vi "UHR-Fleezers Control (host) -Leonardo 04-2018 V1.vi"(0 "Tab Control":T5(tab)=enum."Trap Control (RF)") -> ()   [LabVIEW 2013] (continued)
              tunnel: w2073 -> [_ w2136]
              tunnel: w2071 -> [_ w2135]
              frame False {
              }
              frame True {
                w2131 = FALSE ("Get Point")
                n1369 = local read "Scan lines (y)"() -> (w2140:u64)
                n1370 = local read "Actual MCL Inc (V)"() -> (w2132:dbl)
                n1371 = local read "Scan steps (MCL)"() -> (w2139:u64)
                n1372 = Divide "Y Pix/step"(x=w2135, y=w2140) -> (x/y=w2147:dbl)
                n1373 = Divide "Y V/pix"(x=w2132, y=w2147) -> (x/y=w2146:dbl)
                n1374 = Divide "Y half step offset"(x=w2132, y=2.0) -> (x/y=w2148:dbl)
                n1375 = Divide "X pix/step"(x=w2136, y=w2139) -> (x/y=w2145:dbl)
                n1376 = Negate(x=w2148) -> (-x=w2149:dbl)
                n1377 = local read "Initial Y"() -> (w2155:dbl)
                n1378 = Multiply(x=w2137, y=w2146) -> (x*y=w2156:dbl)
                n1379 = Divide "X half step offset"(x=w2132, y=2.0) -> (x/y=w2142:dbl)
                n1380 = Divide "X V/pix"(x=w2132, y=w2145) -> (x/y=w2144:dbl)
                n1381 = Multiply(x=w2132, y=w2139) -> (x*y=w2151:dbl)
                n1382 = Compound Arithmetic op=ADD(w2149, w2156, w2155) -> (w2133:dbl)
                "Pointer Y (V)" <- w2133
                n1383 = Multiply(x=w2144, y=w2138) -> (x*y=w2153:dbl)
                n1384 = Negate(x=w2142) -> (-x=w2141:dbl)
                n1385 = local read "Initial X"() -> (w2154:dbl)
                n1386 = Negate(x=w2153) -> (-x=w2152:dbl)
                n1387 = Compound Arithmetic op=ADD(w2141, w2151, w2154, w2152) -> (w2134:dbl)
                "Pointer X (V)" <- w2134
                n1388 = Or(x="Set X Only", y="Set Confocal Spot (X-Y)") -> (x .or. y?=w2127:bool)
                n1389 = Or(x="Set Confocal Spot (X-Y)", y="Set Y Only") -> (x .or. y?=w2126:bool)
                n1390 = case shown="True" w2127 {
                  tunnel: w2134 -> [_ w2157]
                  frame False {
                  }
                  frame True {
                    n1391 = property on="AO2" class="Slide (strict)"("Val(Sgnl)"=w2157) -> ()  [unwired: 2 in, 2 out]
                  }
                }
                n1392 = case shown="True" w2126 {
                  tunnel: w2133 -> [_ w2158]
                  frame False {
                  }
                  frame True {
                    n1393 = property on="AO1" class="Slide (strict)"("Val(Sgnl)"=w2158) -> ()  [unwired: 2 in, 2 out]
                  }
                }
                n1394 = local write "Set Confocal Spot (X-Y)"(w2131) -> ()
                n1395 = local write "Set X Only"(w2131) -> ()
                n1396 = local write "Set Y Only"(w2131) -> ()
              }
            }
          }
          frame 3 {
            n1397 = local read "BD 2 Frequency 1 (MHz)"() -> (w2159:dbl)
            n1398 = local read "BD 1 Frequency 1 (MHz)"() -> (w2160:dbl)
            n1399 = local write "Manipulating Trap"(TRUE ("Manipulating Trap")) -> ()
            n1400 = local write "Coords"(T8 {"Horizontal"=0, "Vertical"=0} ("Coords")) -> ()
            n1401 = while {
              tunnel: w2165 -> [w2170]
              tunnel: w2163 -> [w2169]
              tunnel: w2161 -> [w2168]
              tunnel: w2160 -> [w2167]
              tunnel: w2159 -> [w2166]
              stop <- w2171 stop-if-true
              n1402 = event shown="[0] \"Pane\": Mouse Move" {
                selector: _ -> [_ _]
                dyn-events: _ -> [_ _]
                timeout: _ -> [_ _]
                tunnel: ["Force Manip Abort" w2235] -> w2171
                tunnel: w2170 -> [w2178 _]
                tunnel: w2169 -> [w2176 _]
                tunnel: w2168 -> [w2175 _]
                tunnel: w2167 -> [w2174 _]
                tunnel: w2166 -> [w2173 _]
                event Mouse Move {
                  n1403 = event-data() -> ("Time"=w2179:u32, "Coords"=w2180:T8)  [unwired: 3 out]
                  n1404 = Less?(x=w2179, y=w2178) -> (x < y?=w2177:bool)
                  n1405 = case "Makes sure old motion events prior to mouse click aren't used" shown="False" w2177 {
                    tunnel: w2180 -> [w2222 _]
                    tunnel: w2176 -> [w2223 _]
                    tunnel: w2175 -> [w2200 _]
                    tunnel: w2174 -> [w2196 _]
                    tunnel: w2173 -> [w2195 _]
                    frame False {
                      n1406 = Subtract(x=w2222, y=w2223) -> (x-y=w2221:T8)
                      "Coords" <- w2221
                      n1407 = local read "Y RF Frequency Limits (MHz)"() -> (w2181:T16)
                      n1408 = To Double Precision Float(number=w2221) -> (double precision float=w2220:cluster{"Horizontal":dbl, "Vertical":dbl})
                      n1409 = Multiply(x=cluster{"Horizontal":dbl, "Vertical":dbl} {"Horizontal"=-1.0, "Vertical"=1.0}, y="Manipulation Scaling") -> (x*y=w2216:cluster{"Horizontal":dbl, "Vertical":dbl})
                      n1410 = local read "X RF Frequency Limits (MHz)"() -> (w2182:T16)
                      n1411 = Multiply(x=w2220, y=w2216) -> (x*y=w2218:cluster{"Horizontal":dbl, "Vertical":dbl})
                      n1412 = Unbundle By Name(w2218) -> ("Horizontal"=w2213:dbl, "Vertical"=w2217:dbl)
                      n1413 = Unbundle By Name(w2181) -> ("Maximum"=w2184:dbl, "Minimum"=w2183:dbl)
                      n1414 = Boolean To (0,1)(Boolean="Manip. X?") -> (0, 1=w2211:i16)
                      n1415 = Boolean To (0,1)(Boolean="Manip. Y?") -> (0, 1=w2208:i16)
                      n1416 = local read "BD 1 Frequency 2 (MHz)"() -> (w2198:dbl)
                      n1417 = Multiply(x=w2217, y=w2208) -> (x*y=w2210:dbl)
                      n1418 = Multiply(x=w2211, y=w2213) -> (x*y=w2214:dbl)
                      n1419 = local read "BD 2 Frequency 2 (MHz)"() -> (w2197:dbl)
                      n1420 = Unbundle By Name(w2182) -> ("Maximum"=w2186:dbl, "Minimum"=w2185:dbl)
                      n1421 = Add(x=w2195, y=w2210) -> (x+y=w2188:dbl)
                      n1422 = Add(x=w2196, y=w2214) -> (x+y=w2190:dbl)
                      n1423 = In Range and Coerce(upper limit=w2186, x=w2190, lower limit=w2185) -> (coerced(x)=w2189:dbl)  [unwired: 1 out]
                      n1424 = In Range and Coerce(upper limit=w2184, x=w2188, lower limit=w2183) -> (coerced(x)=w2187:dbl)  [unwired: 1 out]
                      n1425 = Subtract(x=w2189, y=w2198) -> (x-y=w2207:dbl)
                      n1426 = Subtract(x=w2187, y=w2197) -> (x-y=w2206:dbl)
                      n1427 = Square(x=w2207) -> (x^2=w2205:dbl)
                      n1428 = Square(x=w2206) -> (x^2=w2204:dbl)
                      n1429 = Add(x=w2205, y=w2204) -> (x+y=w2203:dbl)
                      n1430 = Square Root(x=w2203) -> (sqrt(x)=w2199:dbl)
                      n1431 = In Range and Coerce(upper limit="Limit Max (MHz)", x=w2199, lower limit="Limit Min (MHz)") -> (In Range?=w2192:bool)  [unwired: 1 out]
                      n1432 = Not(x="Limits Enable") -> (.not. x?=w2191:bool)
                      n1433 = Or(x=w2192, y=w2191) -> (x .or. y?=w2193:bool)
                      n1434 = case shown="True" w2193 {
                        tunnel: w2200 -> [_ w2233]
                        tunnel: w2199 -> [_ w2224]
                        tunnel: w2189 -> [_ w2231]
                        tunnel: w2198 -> [_ w2230]
                        tunnel: w2187 -> [_ w2229]
                        tunnel: w2197 -> [_ w2228]
                        tunnel: w2182 -> [_ w2226]
                        tunnel: w2181 -> [_ w2225]
                        frame False {
                        }
                        frame True {
                          n1435 = local read "BD 1 Frequency 3 (MHz)"() -> (w2232:dbl)
                          n1436 = local read "BD 2 Frequency 3 (MHz)"() -> (w2227:dbl)
                          n1437 = local write "Trap Delta (MHz)"(w2224) -> ()
                          n1438 = property on="Initial delta (MHz)" class="DigNum (strict)"("Val(Sgnl)"=w2224) -> ()  [unwired: 2 in, 2 out]
                          n1439 = call "set RF board frequency - interlace.vi"("Board 2 Frequency Limits"=w2225, "Board 1 Frequency Limits"=w2226, "FPGA VI Reference In"=w2233, "Board 2 Frequency 3 (MHz)"=w2227, "Board 1 Frequency 3 (MHz)"=w2232, "Board 2 Frequency 2 (MHz)"=w2228, "Board 2 Frequency 1 (MHz)"=w2229, "Board 1 Frequency 2 (MHz)"=w2230, "Board 1 Frequency 1  (MHz)"=w2231) -> ()  [unwired: 1 in, 2 out]
                          n1440 = local write "BD 2 Frequency 1 (MHz)"(w2229) -> ()
                          n1441 = local write "BD 1 Frequency 1 (MHz)"(w2231) -> ()
                        }
                      }
                    }
                    frame True {
                    }
                  }
                }
                event Mouse Up {
                  n1442 = event-data() -> ("Button"=w2234:u16)  [unwired: 8 out]
                  n1443 = case shown="3" w2234 {
                    tunnel: [FALSE TRUE] -> w2235
                    frame 0, Default {
                    }
                    frame 3 {
                      n1444 = local write "Manipulating Trap"(FALSE ("Manipulating Trap")) -> ()
                    }
                  }
                }
              }
            }
          }
        }
      }
      event Mouse Move {
        n1445 = event-data() -> ()  [unwired: 6 out]
      }
    }
    n1446 = local read "Stop All"() -> (w2056:bool)
    n1447 = node-c288() -> ()  [unwired: 2 out]
  }
  n1448 = node-c288(w51) -> ()  [unwired: 1 out]
  n1449 = node-c288(w101) -> ()  [unwired: 1 out]
  n1450 = node-c288(w108) -> ()  [unwired: 1 out]
  n1451 = node-c288(i64 1 ("Period"), 1 ("Processor")) -> (w194:T25)  [unwired: 2 out]
  n1452 = timed-loop "Acquire Data" {
    tunnel: w59 -> [w2544]
    tunnel: w75 -> [w2543]
    tunnel: [w2574] -> w68
    tunnel: [w2568] -> w67
    timing: w194 -> [_]
    timing-out: [_] -> w193
    tunnel: w92 -> [w2390]
    stop <- "Stop All" stop-if-true
    (unwired) u32 0 ("Number of Elements")
    w2377 = "NI_ChannelName" ("name")
    n1453 = node-c288() -> ()  [unwired: 2 out]
    n1454 = First Call?() -> (First Call?: T/F=w2343:bool)
    n1455 = Or(x="Reset", y=w2343) -> (x .or. y?=w2344:bool)
    n1456 = local read "MCL Tracking"() -> (w2281:bool)
    n1457 = case "Reset data stream" shown="True" w2344 {
      tunnel: w2544 -> [w2694 w2702]
      tunnel: w2543 -> [w2693 w2701]
      tunnel: [w2694 w2696] -> w2279
      tunnel: [w2693 w2695] -> w2539
      frame False {
      }
      frame True {
        w2699 = TRUE ("AI to FIFO")
        n1458 = local write "Overflow (data lost)"(FALSE ("Overflow (data lost)")) -> ()
        n1459 = call "reset FPGA DMA.vi"("error in"=w2701, "FPGA VI Reference In"=w2702) -> ("error out"=w2697:errorcluster, "FPGA VI Reference Out"=w2698:T20)
        n1460 = xnode "Read/Write Control"("FPGA VI Reference In"=w2698, "error in"=w2697, "AI to FIFO"=w2699, "APD to FIFO"=w2699) -> ("FPGA VI Reference Out"=w2696:T20, "error out"=w2695:errorcluster)
      }
    }
    n1461 = Or(x="Start AOD Scan", y="Trap Raster Scan") -> (x .or. y?=w2497:bool)
    n1462 = case "Start AOM raster scan" shown="True" w2497 {
      tunnel: w2279 -> [w3435 w3446]
      tunnel: w2539 -> [w3434 w3445]
      tunnel: [w3435 w3439] -> w2278
      tunnel: [w3434 w3438] -> w2538
      frame False {
      }
      frame True {
        n1463 = case shown="True" "Restart DMA? (AOD)" {
          tunnel: [w3486 w3488] -> w3440
          tunnel: [w3485 w3487] -> w3441
          tunnel: w3446 -> [w3486 w3490]
          tunnel: w3445 -> [w3485 w3489]
          frame False {
          }
          frame True {
            n1464 = local write "Overflow (data lost)"(FALSE ("Overflow (data lost)")) -> ()
            n1465 = call "reset FPGA DMA.vi"("error in"=w3489, "FPGA VI Reference In"=w3490) -> ("error out"=w3487:errorcluster, "FPGA VI Reference Out"=w3488:T20)
          }
        }
        n1466 = local write "Trap Raster Scan"(FALSE ("Trap Raster Scan")) -> ()
        n1467 = case shown="True" "Move MCL Also?" {
          tunnel: w3441 -> [w3450 w3480]
          tunnel: w3440 -> [w3451 w3481]
          tunnel: [w3449 w3484] -> w3439
          tunnel: [w3448 w3483] -> w3438
          tunnel: "Raster to target force?" -> [w3447 w3453]
          frame False {
            w3452 = TRUE ("AI to FIFO")
            n1468 = xnode "Read/Write Control"("FPGA VI Reference In"=w3451, "error in"=w3450, "AI to FIFO"=w3452, "APD to FIFO"=w3452, "Start scan"=w3452, "Raster to target force"=w3447) -> ("FPGA VI Reference Out"=w3449:T20, "error out"=w3448:errorcluster)
          }
          frame True {
            w3477 = FALSE ("1D or 2D Scan?")
            w3482 = TRUE ("AI to FIFO")
            # "Count for MCL loop"
            # "N total cycles"
            # "N steps"
            # "V_int"
            n1469 = local read "Scan Range (nm)"() -> (w3459:dbl)
            n1470 = local read "Number of F/B Scans (AOD)"() -> (w3476:u16)
            n1471 = Sign(1:w3459) -> (0:w3458:dbl)
            n1472 = Compound Arithmetic op=MULTIPLY(w3459, "MCL Step Position Ratio", "MCL/AOM Scale Tweak") -> (w3463:dbl)
            n1473 = Negate(x=w3458) -> (-x=w3455:dbl)
            n1474 = Multiply(x=w3455, y="MCL Step Increment (V_int)") -> (x*y=w3457:dbl)
            n1475 = Divide(x=w3463, y="MCL X Cal (nm/V)") -> (x/y=w3469:dbl)
            n1476 = Multiply(x=32767.0 ("y"), y=w3469) -> (x*y=w3475:dbl)
            n1477 = local read "Total Counts (ticks)"() -> (w3460:u32)
            n1478 = local read "Cycles/step (AOD)"() -> (w3471:u64)
            n1479 = local read "Scan steps (AOD)"() -> (w3472:u64)
            n1480 = Divide(x=w3475, y=10.0) -> (x/y=w3468:dbl)
            n1481 = Divide(x=w3468, y="MCL Step Increment (V_int)") -> (x/y=w3466:dbl)
            n1482 = Absolute Value(x=w3466) -> (abs(x)=w3454:dbl)
            n1483 = Compound Arithmetic op=MULTIPLY(w3472, w3471, w3460) -> (w3467:u64)
            n1484 = local write "wait to reset values"(w3482) -> ()
            n1485 = local write "MCL Scanning"(w3482) -> ()
            n1486 = Divide(x=w3467, y=w3454) -> (x/y=w3464:dbl)
            "MCL Count" <- w3464
            n1487 = xnode "Read/Write Control"("FPGA VI Reference In"=w3481, "error in"=w3480, "Scan steps (MCL)"=w3454, "Number of scans (MCL)"=w3476, "Cycles per step (MCL)"=u64 1, "Scan freq.  increment (MCL)"=w3457, "1D or 2D Scan?"=w3477, "MCL Scan Axis"=w3477, "Cont. Scan (MCL)"=w3477, "MCL count"=w3464) -> ("FPGA VI Reference Out"=w3479:T20, "error out"=w3478:errorcluster)
            n1488 = xnode "Read/Write Control"("FPGA VI Reference In"=w3479, "error in"=w3478, "AI to FIFO"=w3482, "APD to FIFO"=w3482, "Start scan"=w3482, "Start scan (MCL)"=w3482, "Raster to target force"=w3453) -> ("FPGA VI Reference Out"=w3484:T20, "error out"=w3483:errorcluster)
          }
        }
        "Raster Scanning..." <- TRUE ("Scanning...")
      }
    }
    n1489 = And(x="Save scans", y=w2497) -> (x .and. y?=w2537:bool)
    n1490 = Compound Arithmetic op=OR("Start MCL Scan", "Confocal Image", "Confocal Linescan") -> (w2495:bool)
    n1491 = And(x="Save Data (MCL)", y=w2495) -> (x .and. y?=w2536:bool)
    n1492 = case "Start MCL raster scan" shown="True" w2495 {
      tunnel: w2278 -> [w2985 w3000]
      tunnel: w2538 -> [w2984 w2999]
      tunnel: [w2985 w2995] -> w2313
      tunnel: [w2984 w2994] -> w2312
      tunnel: [FALSE w2993] -> w2522
      tunnel: "Start MCL Scan" -> [_ w2988]
      tunnel: "Confocal Image" -> [_ w2987]
      tunnel: "Confocal Linescan" -> [_ _]
      frame False {
      }
      frame True {
        w2993 = TRUE
        n1493 = case shown="True" "Restart DMA? (MCL)" {
          tunnel: [w3045 w3047] -> w2998
          tunnel: [w3044 w3046] -> w2997
          tunnel: w3000 -> [w3045 w3050]
          tunnel: w2999 -> [w3044 w3049]
          frame False {
          }
          frame True {
            n1494 = call "reset FPGA DMA.vi"("error in"=w3049, "FPGA VI Reference In"=w3050) -> ("error out"=w3046:errorcluster, "FPGA VI Reference Out"=w3047:T20)
            n1495 = local write "Overflow (data lost)"(FALSE ("Overflow (data lost)")) -> ()
          }
        }
        n1496 = case shown="False" w2988 {
          selector: w2988 -> [_ w3004]
          tunnel: w2987 -> [w3003 _]
          tunnel: [w3003 w3004] -> w2986
          frame False {
            n1497 = property on="2D or 1D Scan" class="Bool (strict)"("Val(Sgnl)"=w3003) -> ()  [unwired: 2 in, 2 out]
            n1498 = property on="Confocal Image" class="Bool (strict)"("Value"=FALSE ("Start Confocal Map")) -> ()  [unwired: 2 in, 2 out]
          }
          frame True {
          }
        }
        n1499 = local write "MCL Scanning"(w2993) -> ()
        n1500 = local read "AO1"() -> (w2990:dbl)
        n1501 = local read "AO2"() -> (w2989:dbl)
        n1502 = case shown="True" "Center Scan" {
          tunnel: w2998 -> [w3011 w3043]
          tunnel: w2997 -> [w3010 w3042]
          tunnel: [w3009 w3041] -> w2995
          tunnel: [w3008 w3040] -> w2994
          tunnel: [w3006 w3027] -> w2992
          tunnel: [w3005 w3026] -> w2991
          tunnel: w2990 -> [w3006 w3032]
          tunnel: w2989 -> [w3005 w3035]
          tunnel: w2986 -> [_ _]
          frame False {
            w3007 = TRUE ("AI to FIFO")
            n1503 = xnode "Read/Write Control"("FPGA VI Reference In"=w3011, "error in"=w3010, "AI to FIFO"=w3007, "APD to FIFO"=w3007, "Start scan (MCL)"=w3007) -> ("FPGA VI Reference Out"=w3009:T20, "error out"=w3008:errorcluster)
          }
          frame True {
            w3039 = TRUE ("AI to FIFO")
            n1504 = local read "Scan steps (MCL)"() -> (w3018:u64)
            n1505 = local read "Scan lines (y)"() -> (w3014:u64)
            n1506 = local read "Fast Scan Dir"() -> (w3025:bool)
            n1507 = local read "Actual MCL Inc (V)"() -> (w3015:dbl)
            n1508 = Decrement(x=w3014) -> (x-1=w3013:u64)
            n1509 = Decrement(x=w3018) -> (x-1=w3017:u64)
            n1510 = Multiply(x=w3015, y=w3013) -> (x*y=w3012:dbl)
            n1511 = Divide(x=w3012, y=2.0) -> (x/y=w3022:dbl)
            n1512 = Multiply(x=w3015, y=w3017) -> (x*y=w3016:dbl)
            n1513 = Divide(x=w3016, y=2.0) -> (x/y=w3021:dbl)
            n1514 = Select(t=w3021, s=w3025, f=w3022) -> (s? t:f=w3020:dbl)
            n1515 = Select(t=w3022, s=w3025, f=w3021) -> (s? t:f=w3024:dbl)
            n1516 = Subtract(x=w3032, y=w3024) -> (x-y=w3023:dbl)
            n1517 = Subtract(x=w3035, y=w3020) -> (x-y=w3019:dbl)
            n1518 = local read "2D or 1D Scan"() -> (w3037:bool)
            n1519 = Not(x=w3025) -> (.not. x?=w3031:bool)
            n1520 = Not(x=w3037) -> (.not. x?=w3033:bool)
            n1521 = And(x=w3025, y=w3033) -> (x .and. y?=w3034:bool)
            n1522 = And(x=w3033, y=w3031) -> (x .and. y?=w3036:bool)
            n1523 = Select(t=w3035, s=w3036, f=w3019) -> (s? t:f=w3026:dbl)
            n1524 = Select(t=w3032, s=w3034, f=w3023) -> (s? t:f=w3027:dbl)
            n1525 = call "Volt to I16.vi"("Voltage In"=w3027) -> ("I16 Voltage Out"=w3030:i16)
            n1526 = call "Volt to I16.vi"("Voltage In"=w3026) -> ("I16 Voltage Out"=w3029:i16)
            n1527 = xnode "Read/Write Control"("FPGA VI Reference In"=w3043, "error in"=w3042, "AI to FIFO"=w3039, "APD to FIFO"=w3039, "Start scan (MCL)"=w3039, "AO1 (Y)"=w3030, "AO2 (X)"=w3029) -> ("FPGA VI Reference Out"=w3041:T20, "error out"=w3040:errorcluster)
          }
        }
        "Initial Y" <- w2992
        "Initial X" <- w2991
        "wait to reset values" <- w2993
      }
    }
    n1528 = local read "Trap Pos Elements/DMA read"() -> (w2386:u32)
    n1529 = local read "Trap AI Elements/DMA read"() -> (w2311:u32)
    n1530 = local read "APD Elements/DMA read"() -> (w2425:u32)
    n1531 = local read "Trap AI FIFO Depth"() -> (w2584:u32)
    n1532 = xnode "Invoke Method"("FPGA VI Reference In"=w2313, "error in"=w2312, "Number of Elements"=w2386, "Timeout (ms)"=-1) -> ("Data"=w2350:u16[], "Elements Remaining"=→"Trap Pos FIFO El Remaining":u32)  [unwired: 2 out]
    n1533 = xnode "Invoke Method"("FPGA VI Reference In"=w2313, "error in"=w2312, "Number of Elements"=w2311, "Timeout (ms)"=-1 ("Timeout")) -> ("FPGA VI Reference Out"=w2282:T20, "error out"=w2314:errorcluster, "Data"=w2310:i16[], "Elements Remaining"=w2315:u32)
    "Trap AI FIFO El. Rem." <- w2315
    n1534 = xnode "Get APD Data"("FPGA VI Reference In"=w2313, "error in"=w2312, "Number of Elements"=w2425, "Timeout (ms)"=-1) -> ("Data"=w2424:u32[], "Elements Remaining"=→"APD FIFO Elements Remaining":u32)  [unwired: 2 out]
    n1535 = Subtract(x=w2584, y=w2311) -> (x-y=w2583:u32)
    n1536 = Decimate 1D Array(w2350) -> (w2347:u16[], w2349:u16[], w2348:u16[])
    n1537 = Divide(x=w2315, y=w2583) -> (x/y=w2582:dbl)
    "Buffer Status" <- w2582
    n1538 = To Unsigned Long Integer(number=w2347) -> (unsigned 32bit integer=w2346:u32[])
    n1539 = Join Numbers(hi=w2349, lo=w2348) -> ((hi.lo)=w2345:u32[])
    n1540 = Equal?(x=w2582, y=1.0) -> (x = y?=w2580:bool)
    n1541 = Join Numbers(hi=w2346, lo=w2345) -> ((hi.lo)=w2339:u64[])
    n1542 = call "IR AOM word to freq - vec.vi"("Frequency Word In (double vec)"=w2339) -> ("Frequency Out"=w2385:dbl[])
    n1543 = case "Alert buffer overflow" shown="True" w2580 {
      frame False {
      }
      frame True {
        n1544 = call <vilib>:"Beep.vi"() -> ()  [unwired: 3 in, 9 out]
        "Overflow (data lost)" <- TRUE ("Overflow (data lost)")
      }
    }
    n1545 = Decimate 1D Array(w2385) -> (w2384:dbl[], w2383:dbl[])
    n1546 = Array Size(array=w2310) -> (size(s)=→"Waveform Chart":i32)
    n1547 = Build Array(w2384, w2383) -> (w2382:dbl[][])
    n1548 = local read "Trap Sets"() -> (w2457:u32)
    n1549 = case "Deinterlace trap data, average down PSD" shown="2" w2457 {
      tunnel: w2310 -> [w3080 w3145]
      tunnel: [w3077 w3142] -> w2450
      tunnel: [w3080 w3144] -> w2342
      tunnel: "Detector Type" -> [w3079 w3140]
      tunnel: [w3078 w3143] -> w2449
      tunnel: [w3076 w3141] -> w2555
      frame 1, Default {
        n1550 = Divide(x=w3080, y=3276.7) -> (x/y=w3081:dbl[])
        n1551 = Decimate 1D Array(w3081) -> (w3090:dbl[], w3089:dbl[], w3088:dbl[], w3087:dbl[], w3086:dbl[], w3085:dbl[], w3084:dbl[], w3083:dbl[])
        n1552 = case shown="\"IR-QPD + PSD + FB-QPD position\"" w3079 {
          tunnel: w3090 -> [w3114 w3139]
          tunnel: w3089 -> [w3113 w3138]
          tunnel: w3088 -> [w3098 w3116]
          tunnel: w3087 -> [w3099 w3126]
          tunnel: w3086 -> [w3112 w3137]
          tunnel: w3085 -> [w3111 w3136]
          tunnel: w3084 -> [w3095 w3117]
          tunnel: w3083 -> [w3094 w3115]
          tunnel: [w3093 w3123] -> w3078
          tunnel: [w3092 w3122] -> w3077
          tunnel: [w3091 w3121] -> w3076
          frame "IR-QPD + PSD + FB-QPD", Default {
            w3091 = 0  # Channel pattern
            n1553 = Divide(x=w3114, y=w3099) -> (x/y=w3101:dbl[])
            n1554 = Divide(x=w3113, y=w3099) -> (x/y=w3100:dbl[])
            n1555 = Divide(x=w3112, y=w3095) -> (x/y=w3097:dbl[])
            n1556 = Divide(x=w3111, y=w3094) -> (x/y=w3096:dbl[])
            n1557 = Build Array(w3101, w3100, w3099, w3098, w3097, w3096, w3095, w3094) -> (w3092:dbl[][])
            n1558 = Bundle("T1 Y", "T1 X", "T1 Sum", "FB Sum", "PSD Y", "PSD X", "PSD Y Sum", "PSD X Sum") -> (w3110:T42)  [unwired: 1 out]
            n1559 = Cluster To Array(cluster=w3110) -> (array=w3093:string[])
          }
          frame "IR-QPD + PSD + FB-QPD position" {
            w3121 = 3  # Channel pattern
            n1560 = Negate(x=w3117) -> (-x=w3118:dbl[])
            n1561 = Divide(x=w3139, y=w3126) -> (x/y=w3128:dbl[])
            n1562 = Divide(x=w3138, y=w3126) -> (x/y=w3127:dbl[])
            n1563 = Divide(x=w3137, y=w3117) -> (x/y=w3125:dbl[])
            n1564 = Divide(x=w3136, y=w3118) -> (x/y=w3124:dbl[])
            n1565 = Build Array(w3128, w3127, w3126, w3115, w3116, w3125, w3124, w3117) -> (w3122:dbl[][])
            n1566 = Bundle("T1 Y", "T1 X", "T1 Sum", "FB X", "FB Sum", "PSD Y", "PSD X", "PSD Y Sum") -> (w3135:T42)  [unwired: 1 out]
            n1567 = Cluster To Array(cluster=w3135) -> (array=w3123:string[])
          }
        }
      }
      frame 2 {
        n1568 = case shown="\"UCB Fleezers 052511\"" w3140 {
          tunnel: w3145 -> [w3207 w3274 w3313 w3413]
          tunnel: [w3146 w3266 w3309 w3344] -> w3144
          tunnel: [w3173 w3257 w3311 w3391] -> w3143
          tunnel: [w3172 w3221 w3302 w3358] -> w3142
          tunnel: [w3166 w3256 w3343 w3389] -> w3141
          frame "IR-QPD + PSD + FB-QPD", Default {
            w3166 = 1  # Channel pattern
            # "time average x2 the 4th signal and the 4 psd signals (detection laser)"
            # "deinterlace 3 signals from qpd"
            n1569 = Decimate 1D Array(w3207) -> (w3206:i16[], w3205:i16[], w3171:i16[], w3204:i16[], w3194:i16[], w3192:i16[], w3191:i16[], w3189:i16[])
            n1570 = call "downsample 1D array - double.vi"("Ave N"=2.0, "Array In"=w3194) -> ("Array Out"=w3193:dbl[])  [unwired: 1 out]
            n1571 = call "downsample 1D array - double.vi"("Ave N"=2.0, "Array In"=w3189) -> ("Array Out"=w3188:dbl[])  [unwired: 1 out]
            n1572 = call "downsample 1D array - double.vi"("Ave N"=2.0, "Array In"=w3191) -> ("Array Out"=w3190:dbl[])  [unwired: 1 out]
            n1573 = call "downsample 1D array - double.vi"("Ave N"=2.0, "Array In"=w3192) -> ("Array Out"=w3174:dbl[])  [unwired: 1 out]
            n1574 = Decimate 1D Array(w3206) -> (w3203:i16[], w3175:i16[])
            n1575 = Decimate 1D Array(w3205) -> (w3202:i16[], w3200:i16[])
            n1576 = Decimate 1D Array(w3204) -> (w3201:i16[], w3199:i16[])
            n1577 = Decimate 1D Array(w3171) -> (w3170:i16[], w3169:i16[])
            n1578 = Interleave 1D Arrays(w3203, w3202, w3201, w3175, w3200, w3199, w3170, w3169, w3193, w3174, w3190, w3188) -> (w3187:dbl[])
            n1579 = To Word Integer(number=w3187) -> (16bit integer=w3146:i16[])
            n1580 = Divide(x=w3187, y=3276.7) -> (x/y=w3186:dbl[])
            n1581 = Decimate 1D Array(w3186) -> (w3185:dbl[], w3184:dbl[], w3183:dbl[], w3182:dbl[], w3181:dbl[], w3180:dbl[], w3168:dbl[], w3167:dbl[], w3179:dbl[], w3178:dbl[], w3177:dbl[], w3176:dbl[])
            n1582 = Divide(x=w3185, y=w3183) -> (x/y=w3153:dbl[])
            n1583 = Divide(x=w3184, y=w3183) -> (x/y=w3152:dbl[])
            n1584 = Divide(x=w3182, y=w3180) -> (x/y=w3151:dbl[])
            n1585 = Divide(x=w3181, y=w3180) -> (x/y=w3150:dbl[])
            n1586 = Divide(x=w3179, y=w3177) -> (x/y=w3149:dbl[])
            n1587 = Divide(x=w3178, y=w3176) -> (x/y=w3148:dbl[])
            n1588 = Bundle("T1 Y", "T1 X", "T1 Sum", "T2 Y", "T2 X", "T2 Sum", "T1 FB Sum", "T2 FB Sum", "PSD Y", "PSD X", "PSD Y Sum", "PSD X Sum") -> (w3154:T43)  [unwired: 1 out]
            n1589 = Build Array(w3153, w3152, w3183, w3151, w3150, w3180, w3168, w3167, w3149, w3148, w3177, w3176) -> (w3172:dbl[][])
            n1590 = Cluster To Array(cluster=w3154) -> (array=w3173:string[])
          }
          frame "IR-QPD + PSD + FB-QPD X position" {
            w3256 = 2  # Channel pattern
            # "convert\nADC numbers\nto volts"
            # "time average x2 the 3 psd signals (detection laser)"
            # "deinterlace 3 signals from qpds"
            n1591 = Decimate 1D Array(w3274) -> (w3273:i16[], w3272:i16[], w3209:i16[], w3210:i16[], w3219:i16[], w3216:i16[], w3213:i16[], w3244:i16[])
            n1592 = Decimate 1D Array(w3273) -> (w3271:i16[], w3258:i16[])
            n1593 = call "downsample 1D array - I16.vi"("Ave N"=2.0, "Array In"=w3219) -> ("Array Out"=w3217:i16[])  [unwired: 1 in]
            n1594 = call "downsample 1D array - I16.vi"("Ave N"=2.0, "Array In"=w3216) -> ("Array Out"=w3214:i16[])  [unwired: 1 in]
            n1595 = Decimate 1D Array(w3272) -> (w3270:i16[], w3268:i16[])
            n1596 = Decimate 1D Array(w3210) -> (w3269:i16[], w3267:i16[])
            n1597 = Decimate 1D Array(w3244) -> (w3243:i16[], w3241:i16[])
            n1598 = Decimate 1D Array(w3209) -> (w3242:i16[], w3240:i16[])
            n1599 = call "downsample 1D array - I16.vi"("Ave N"=2.0, "Array In"=w3213) -> ("Array Out"=w3211:i16[])  [unwired: 1 in]
            n1600 = Interleave 1D Arrays(w3271, w3270, w3269, w3258, w3268, w3267, w3243, w3242, w3241, w3240, w3217, w3214, w3211) -> (w3266:i16[])
            n1601 = Divide(x=w3266, y=3276.7) -> (x/y=w3265:dbl[])
            n1602 = Decimate 1D Array(w3265) -> (w3264:dbl[], w3263:dbl[], w3262:dbl[], w3261:dbl[], w3260:dbl[], w3259:dbl[], w3232:dbl[], w3230:dbl[], w3229:dbl[], w3227:dbl[], w3226:dbl[], w3225:dbl[], w3222:dbl[])
            n1603 = Divide(x=w3264, y=w3262) -> (x/y=w3248:dbl[])
            n1604 = Divide(x=w3263, y=w3262) -> (x/y=w3247:dbl[])
            n1605 = Divide(x=w3261, y=w3259) -> (x/y=w3246:dbl[])
            n1606 = Divide(x=w3260, y=w3259) -> (x/y=w3245:dbl[])
            n1607 = Divide(x=w3232, y=w3230) -> (x/y=w3231:dbl[])
            n1608 = Divide(x=w3229, y=w3227) -> (x/y=w3228:dbl[])
            n1609 = Divide(x=w3226, y=w3222) -> (x/y=w3224:dbl[])
            n1610 = Negate(x=w3222) -> (-x=w3220:dbl[])
            n1611 = Divide(x=w3225, y=w3220) -> (x/y=w3223:dbl[])
            n1612 = Bundle("T1 Y", "T1 X", "T1 Sum", "T2 Y", "T2 X", "T2 Sum", "T1 FB X", "T1 FB Sum", "T2 FB X", "T2 FB Sum", "PSD Y", "PSD X", "PSD Y Sum") -> (w3249:T44)  [unwired: 1 out]
            n1613 = Build Array(w3248, w3247, w3262, w3246, w3245, w3259, w3231, w3230, w3228, w3227, w3224, w3223, w3222) -> (w3221:dbl[][])
            n1614 = Cluster To Array(cluster=w3249) -> (array=w3257:string[])
          }
          frame "UCB Fleezers 052511" {
            w3343 = 2  # Channel pattern
            n1615 = Select(t=i16 -1, s="Negate X signals", f=i16 1) -> (s? t:f=w3283:i16)
            n1616 = Decimate 1D Array(w3313) -> (w3284:i16[], w3285:i16[], w3296:i16[], w3312:i16[], w3281:i16[], w3279:i16[], w3277:i16[], w3293:i16[])
            n1617 = Multiply(x=w3283, y=w3285) -> (x*y=w3282:i16[])
            n1618 = Decimate 1D Array(w3284) -> (w3341:i16[], w3331:i16[])
            n1619 = Decimate 1D Array(w3282) -> (w3340:i16[], w3339:i16[])
            n1620 = Decimate 1D Array(w3296) -> (w3290:i16[], w3289:i16[])
            n1621 = Decimate 1D Array(w3312) -> (w3295:i16[], w3294:i16[])
            n1622 = Decimate 1D Array(w3279) -> (w3278:i16[])  [unwired: 1 out]
            n1623 = Decimate 1D Array(w3293) -> (w3292:i16[], w3291:i16[])
            n1624 = Decimate 1D Array(w3277) -> (w3276:i16[])  [unwired: 1 out]
            n1625 = Decimate 1D Array(w3281) -> (w3280:i16[])  [unwired: 1 out]
            n1626 = Interleave 1D Arrays(w3341, w3340, w3295, w3331, w3339, w3294, w3292, w3290, w3291, w3289, w3280, w3278, w3276) -> (w3309:i16[])
            n1627 = Divide(x=w3309, y=3276.7) -> (x/y=w3338:dbl[])
            n1628 = Decimate 1D Array(w3338) -> (w3337:dbl[], w3336:dbl[], w3335:dbl[], w3334:dbl[], w3333:dbl[], w3332:dbl[], w3308:dbl[], w3306:dbl[], w3305:dbl[], w3303:dbl[], w3301:dbl[], w3298:dbl[], w3299:dbl[])
            n1629 = Divide(x=w3337, y=w3335) -> (x/y=w3318:dbl[])
            n1630 = Divide(x=w3336, y=w3335) -> (x/y=w3317:dbl[])
            n1631 = Divide(x=w3334, y=w3332) -> (x/y=w3316:dbl[])
            n1632 = Divide(x=w3333, y=w3332) -> (x/y=w3315:dbl[])
            n1633 = Divide(x=w3308, y=w3306) -> (x/y=w3307:dbl[])
            n1634 = Divide(x=w3305, y=w3303) -> (x/y=w3304:dbl[])
            n1635 = Divide(x=w3301, y=w3299) -> (x/y=w3300:dbl[])
            n1636 = Divide(x=w3298, y=w3299) -> (x/y=w3297:dbl[])
            n1637 = Build Array(w3318, w3317, w3335, w3316, w3315, w3332, w3307, w3306, w3304, w3303, w3300, w3297, w3299) -> (w3302:dbl[][])
            n1638 = Bundle("T1 Y", "T1 X", "T1 Sum", "T2 Y", "T2 X", "T2 Sum", "T1 FB X", "T2 FB Sum", "T2 FB X", "T2 FB Sum", "PSD Y", "PSD X", "PSD Sum") -> (w3319:T44)  [unwired: 1 out]
            n1639 = Cluster To Array(cluster=w3319) -> (array=w3311:string[])
          }
          frame "IR-QPD + PSD + FB-QPD XY positions" {
            w3389 = 4  # Channel pattern
            # "time average x2 the 3 psd signals (detection laser)"
            # "deinterlace 3 signals from qpds"
            n1640 = Decimate 1D Array(w3413) -> (w3412:i16[], w3411:i16[], w3390:i16[], w3410:i16[], w3356:i16[], w3402:i16[], w3401:i16[], w3378:i16[])
            n1641 = Decimate 1D Array "QPD Y"(w3412) -> (w3409:i16[], w3392:i16[])
            n1642 = call "downsample 1D array - double.vi"("Ave N"=2.0, "Array In"=w3402) -> ("Array Out"=w3377:dbl[])  [unwired: 1 out]
            n1643 = call "downsample 1D array - double.vi"("Ave N"=2.0, "Array In"=w3401) -> ("Array Out"=w3376:dbl[])  [unwired: 1 out]
            n1644 = Decimate 1D Array "Feedback Sum"(w3390) -> (w3374:i16[], w3372:i16[])
            n1645 = Decimate 1D Array "Feedback Y"(w3356) -> (w3355:i16[], w3354:i16[])
            n1646 = Decimate 1D Array "Feedback X"(w3378) -> (w3375:i16[], w3373:i16[])
            n1647 = Decimate 1D Array "QPD Sum"(w3410) -> (w3407:i16[], w3405:i16[])
            n1648 = Decimate 1D Array "QPD X"(w3411) -> (w3408:i16[], w3406:i16[])
            n1649 = Interleave 1D Arrays(w3409, w3408, w3407, w3392, w3406, w3405, w3355, w3375, w3374, w3354, w3373, w3372, w3377, w3376) -> (w3400:dbl[])
            n1650 = To Word Integer(number=w3400) -> (16bit integer=w3344:i16[])
            n1651 = Divide(x=w3400, y=3276.7) -> (x/y=w3399:dbl[])
            n1652 = Decimate 1D Array(w3399) -> (w3398:dbl[], w3397:dbl[], w3396:dbl[], w3395:dbl[], w3394:dbl[], w3393:dbl[], w3351:dbl[], w3365:dbl[], w3349:dbl[], w3350:dbl[], w3363:dbl[], w3347:dbl[], w3361:dbl[], w3359:dbl[])
            n1653 = Divide(x=w3398, y=w3396) -> (x/y=w3382:dbl[])
            n1654 = Divide(x=w3397, y=w3396) -> (x/y=w3381:dbl[])
            n1655 = Divide(x=w3395, y=w3393) -> (x/y=w3380:dbl[])
            n1656 = Divide(x=w3394, y=w3393) -> (x/y=w3379:dbl[])
            n1657 = Divide(x=w3351, y=w3349) -> (x/y=w3348:dbl[])
            n1658 = Divide(x=w3365, y=w3349) -> (x/y=w3364:dbl[])
            n1659 = Divide(x=w3350, y=w3347) -> (x/y=w3346:dbl[])
            n1660 = Divide(x=w3363, y=w3347) -> (x/y=w3362:dbl[])
            n1661 = Negate(x=w3359) -> (-x=w3357:dbl[])
            n1662 = Divide(x=w3361, y=w3357) -> (x/y=w3360:dbl[])
            n1663 = Bundle("T1 Y", "T1 X", "T1 Sum", "T2 Y", "T2 X", "T2 Sum", "T1 FB Y", "T1 FB X", "T1 FB Sum", "T2 FB Y", "T2 FB X", "T2 FB Sum", "PSD X", "PSD Y Sum") -> (w3345:T45)  [unwired: 1 out]
            n1664 = Build Array(w3382, w3381, w3396, w3380, w3379, w3393, w3348, w3364, w3349, w3346, w3362, w3347, w3360, w3359) -> (w3358:dbl[][])
            n1665 = Cluster To Array(cluster=w3345) -> (array=w3391:string[])
          }
        }
      }
    }
    "AI labels" <- w2449
    n1666 = xnode "Read/Write Control"("FPGA VI Reference In"=w2282) -> ("FPGA VI Reference Out"=w2275:T20, "BD1 Frequency Out 1"=w2296:u64)  [unwired: 1 in, 1 out]
    n1667 = local read "BD 1 Frequency 2 (MHz)"() -> (w2287:dbl)
    n1668 = To Double Precision Float(number=w2296) -> (double precision float=w2293:dbl)
    n1669 = Multiply(x=49125000.0, y=6.0) -> (x*y=w2292:dbl)
    n1670 = Multiply(x=w2293, y=w2292) -> (x*y=w2290:dbl)
    n1671 = Scale By Power Of 2(n=-48, x=w2290) -> (x*2^n=w2289:dbl)
    n1672 = local read "Dynamic Force FB"() -> (w2286:bool)
    n1673 = local read "Trap Pos. FB ON"() -> (w2285:bool)
    n1674 = Divide(x=w2289, y=1000000.0) -> (x/y=w2280:dbl)
    n1675 = case shown="True" w2281 {
      tunnel: w2280 -> [_ w2671]
      tunnel: w2278 -> [_ w2658]
      frame False {
      }
      frame True {
        n1676 = local read "AOM X Cal (nm/MHz)"() -> (w2668:dbl)
        n1677 = local read "Zero T1 position"() -> (w2670:dbl)
        n1678 = Subtract(x=w2671, y=w2670) -> (x-y=w2669:dbl)
        n1679 = Multiply(x=w2669, y=w2668) -> (x*y=w2667:dbl)
        n1680 = local read "MCL X Cal (nm/V)"() -> (w2664:dbl)
        n1681 = Multiply(x=w2667, y="Tracking factor") -> (x*y=w2665:dbl)
        n1682 = local read "Zero MCL x position"() -> (w2663:dbl)
        n1683 = Divide(x=w2665, y=w2664) -> (x/y=w2662:dbl)
        n1684 = Add(x=w2663, y=w2662) -> (x+y=w2655:dbl)
        "Current MCL (V)" <- w2655
        n1685 = Multiply(x=w2655, y=32767.0) -> (x*y=w2659:dbl)
        n1686 = Divide(x=w2659, y=10.0) -> (x/y=w2656:dbl)
        n1687 = To Word Integer(number=w2656) -> (16bit integer=w2657:i16)
        n1688 = xnode "Read/Write Control"("FPGA VI Reference In"=w2658, "AO2 (X)"=w2657) -> ()  [unwired: 1 in, 2 out]
      }
    }
    n1689 = Subtract(x=w2287, y=w2280) -> (x-y=w2276:dbl)
    "Current deltaFreq" <- w2276
    n1690 = Compound Arithmetic op=AND(w2286, w2285, "Real time offset \ncorrection for setpoint") -> (w2283:bool)
    n1691 = case shown="True" w2283 {
      tunnel: w2276 -> [_ w2674]
      tunnel: w2275 -> [_ w2673]
      frame False {
      }
      frame True {
        n1692 = local read "T1 kappa_x (pN/nm)"() -> (w2682:dbl)
        n1693 = local read "T1 alpha_x (nm/V)"() -> (w2683:dbl)
        n1694 = local read "Negate offset difference"() -> (w2684:bool)
        n1695 = local read "Offset file step size"() -> (w2692:dbl)
        n1696 = Multiply(x="Target Force (pN)", y=2.0) -> (x*y=w2680:dbl)
        n1697 = local read "Setpoint offset\nCorrection values"() -> (w2689:dbl[])
        n1698 = Divide(x=w2674, y=w2692) -> (x/y=w2691:dbl)
        n1699 = Select(t=-1, s=w2684, f=1) -> (s? t:f=w2685:i32)
        n1700 = To Long Integer(number=w2691) -> (32bit integer=w2690:i32)
        n1701 = Multiply(x=w2683, y=w2682) -> (x*y=w2679:dbl)
        n1702 = Divide(x=w2680, y=w2679) -> (x/y=w2678:dbl)
        n1703 = Index Array(array=w2689, index=w2690) -> (element=w2688:dbl)
        n1704 = Multiply(x=w2685, y=w2688) -> (x*y=w2677:dbl)
        n1705 = Add(x=w2678, y=w2677) -> (x+y=w2676:dbl)
        n1706 = To Fixed-Point(number=w2676) -> (fixed-point=w2672:fxp<+/-,16,1>)  [unwired: 1 in]
        "Actual setpoint" <- w2672
        n1707 = xnode "Read/Write Control"("FPGA VI Reference In"=w2673, "Trap Pos. FB SP"=w2672) -> ()  [unwired: 1 in, 2 out]
      }
    }
    n1708 = case shown="True" "Take full offset\n data for display" {
      tunnel: [w2641 w2647] -> w2474
      tunnel: [w2640 w2646] -> w2472
      tunnel: w2276 -> [_ w2653]
      frame False {
        n1709 = Divide(x="T2 offset_x (mV)", y=1000.0) -> (x/y=w2640:dbl)
        n1710 = Divide(x="T1 offset_x (mV)", y=1000.0) -> (x/y=w2641:dbl)
      }
      frame True {
        n1711 = local read "Offset Values"() -> (w2654:T14)
        n1712 = local read "Offset file step size"() -> (w2652:dbl)
        n1713 = Unbundle By Name(w2654) -> ("Trap 1X offset"=w2649:dbl[], "Trap 2X offset"=w2648:dbl[])
        n1714 = Divide(x=w2653, y=w2652) -> (x/y=w2651:dbl)
        n1715 = To Long Integer(number=w2651) -> (32bit integer=w2650:i32)
        n1716 = Index Array(array=w2649, index=w2650) -> (element=w2647:dbl)
        n1717 = Index Array(array=w2648, index=w2650) -> (element=w2646:dbl)
      }
    }
    n1718 = Decimate 1D Array(w2424) -> (w2447:u32[], w2392:u32[])
    n1719 = local read "DMA Update Period (s)"() -> (w2458:dbl)
    n1720 = local read "BD 1 Frequency 2 (MHz)"() -> (w2334:dbl)
    n1721 = local read "BD 1 Frequency 1 (MHz)"() -> (w2335:dbl)
    n1722 = Build Array(w2447, w2392) -> (w2519:u32[][])
    n1723 = local read "Data Period (s)"() -> (w2437:dbl)
    n1724 = Decimate 1D Array(w2342) -> (w2365:i16[], w2364:i16[], w2362:i16[], w2361:i16[])  [unwired: 9 out]
    n1725 = To Double Precision Float(number=w2519) -> (double precision float=w2520:dbl[][])
    n1726 = local read "APD Integration Time (s)"() -> (w2405:dbl)
    n1727 = Divide(x=w2365, y=w2364) -> (x/y=w2366:dbl[])
    n1728 = Divide(x=w2362, y=w2361) -> (x/y=w2363:dbl[])
    n1729 = feedback #1(0.0) -> (w2379:dbl)
    n1730 = Add(x=w2458, y=w2379) -> (x+y=w2557:dbl)
    n1731 = feedback-in #1(w2557) -> ()
    n1732 = local read "AOM X Cal (nm/MHz)"() -> (w2332:dbl)
    n1733 = To Time Stamp(1:w2379) -> (0:w2378:timestamp)
    n1734 = Split 1D Array(array=w2366, index="N El. to Ave.") -> (second subarray=w2369:dbl[])  [unwired: 1 out]
    n1735 = Split 1D Array(array=w2363, index="N El. to Ave.") -> (second subarray=w2368:dbl[])  [unwired: 1 out]
    n1736 = local read "Trap X AI1 (DMA)"() -> (w2367:T13)
    n1737 = Multiply(x=w2437, y="Trap Disp. Downsample") -> (x*y=w2380:dbl)
    "Display Period (s)" <- w2380
    n1738 = Bundle("BD 1 Frequency 1 (MHz)"=w2335, "BD 1 Frequency 2 (MHz)"=w2334) -> (w2336:T46)  [unwired: 1 out]
    n1739 = for "Trap AI" {
      tunnel: [w3075] -> w2551 mode=indexing
      tunnel: w2378 -> [w3065]
      tunnel: "Trap Disp. Downsample" -> [w3073]
      tunnel: w2450 -> [w3071] mode=indexing
      tunnel: w2437 -> [w3070]
      tunnel: w2449 -> [w3069] mode=indexing
      tunnel: w2377 -> [w3068]
      tunnel: [w3067] -> w2416 mode=indexing
      tunnel: w2380 -> [w3066]
      n1740 = Bundle By Name("Y"=w3071, "dt"=w3070) -> (w3072:waveform(dbl))  [unwired: 1 out]
      n1741 = Set Waveform Attribute(5:w3069, 6:w3068, 7:w3072) -> (3:w3067:waveform(dbl))  [unwired: 1 in, 2 out]
      n1742 = call "downsample 1D array - double.vi"("Ave N"=w3073, "Array In"=w3071) -> ("Array Out"=w3074:dbl[])  [unwired: 1 out]
      n1743 = Bundle By Name(cluster=w3067, "t0"=w3065, "Y"=w3074, "dt"=w3066) -> (w3075:waveform(dbl))
    }
    n1744 = call-poly <vilib>:"Mean.vi"("X"=w2368) -> ("mean"=w2356:dbl)  [unwired: 1 out]
    n1745 = call-poly <vilib>:"Mean.vi"("X"=w2369) -> ("mean"=w2357:dbl)  [unwired: 1 out]
    n1746 = Cluster To Array(cluster=w2336) -> (array=w2333:dbl[])
    n1747 = Reciprocal(x=w2380) -> (1/x=→"Trap Disp. Freq. (Hz)":dbl)
    n1748 = local read "Data points/scans (MCL)"() -> (w2531:dbl)
    n1749 = To Fixed-Point(number=w2356) -> (fixed-point=w2354:fxp<+/-,16,1>)  [unwired: 1 in]
    n1750 = To Fixed-Point(number=w2357) -> (fixed-point=w2355:fxp<+/-,16,1>)  [unwired: 1 in]
    n1751 = Bundle("Trap 1 Pos.", "Trap 2 Pos.") -> (w2376:cluster{string, string})  [unwired: 1 out]
    n1752 = Bundle By Name(cluster=w2367, "Set 1"=w2355, "Set 2"=w2354) -> (→"Trap X AI1 (DMA)":T13)
    n1753 = Cluster To Array(cluster=w2376) -> (array=w2373:string[])
    n1754 = for "Trap Position" {
      tunnel: w2382 -> [w2715] mode=indexing
      tunnel: "Trap Disp. Downsample" -> [w2714]
      tunnel: w2380 -> [w2712]
      tunnel: w2378 -> [w2711]
      tunnel: w2377 -> [w2709]
      tunnel: w2373 -> [w2708] mode=indexing
      tunnel: [w2707] -> w2331 mode=indexing
      tunnel: w2333 -> [w2705] mode=indexing
      tunnel: w2332 -> [w2703]
      n1755 = call "downsample 1D array - double.vi"("Ave N"=w2714, "Array In"=w2715) -> ("Array Out"=w2713:dbl[])  [unwired: 1 out]
      n1756 = Subtract(x=w2713, y=w2705) -> (x-y=w2706:dbl[])
      n1757 = Multiply(x=w2703, y=w2706) -> (x*y=w2704:dbl[])
      n1758 = Bundle By Name("Y"=w2704, "dt"=w2712, "t0"=w2711) -> (w2710:waveform(dbl))  [unwired: 1 out]
      n1759 = Set Waveform Attribute(5:w2708, 6:w2709, 7:w2710) -> (3:w2707:waveform(dbl))  [unwired: 1 in, 2 out]
    }
    "Trap Positions" <- w2331
    n1760 = Bundle("APD 1", "APD 2") -> (w2550:cluster{string, string})  [unwired: 1 out]
    n1761 = Cluster To Array(cluster=w2550) -> (array=w2547:string[])
    n1762 = for "APD" {
      tunnel: w2520 -> [w3054] mode=indexing
      tunnel: w2405 -> [w3062]
      tunnel: [w3058] -> w2412 mode=indexing
      tunnel: "APD Disp. Scale" -> [w3059]
      tunnel: w2377 -> [w3057]
      tunnel: w2547 -> [w3056] mode=indexing
      tunnel: "APD Disp. Downsample" -> [w3052]
      tunnel: [w3055] -> w2546
      tunnel: w2378 -> [w3051]
      n1763 = call "integrate 1D array interval - double.vi"("Ave N"=w3052, "Array In"=w3054) -> ("Array Out"=w3053:dbl[])  [unwired: 1 out]
      n1764 = Multiply(x=w3062, y=w3052) -> (x*y=w3055:dbl)
      n1765 = Divide(x=w3053, y=w3059) -> (x/y=w3060:dbl[])
      n1766 = Bundle By Name("t0"=w3051, "Y"=w3060, "dt"=w3055) -> (w3061:waveform(dbl))  [unwired: 1 out]
      n1767 = Set Waveform Attribute(5:w3056, 6:w3057, 7:w3061) -> (3:w3058:waveform(dbl))  [unwired: 1 in, 2 out]
    }
    "APD Display Period (s)" <- w2546
    n1768 = Reciprocal(x=w2546) -> (1/x=→"APD Display Freq. (Hz)":dbl)
    n1769 = local read "Display Period (s)"() -> (w2436:dbl)
    n1770 = Increment(x=w2531) -> (x+1=w2532:dbl)
    n1771 = Index Array(array=w2331, index=0) -> (element=w2329:waveform(dbl))
    n1772 = To Double Precision Float(number=w2447) -> (double precision float=w2446:dbl[])
    n1773 = feedback #2(w2532) -> (w2535:dbl)
    n1774 = Select(t=0, s=w2522, f=w2535) -> (s? t:f=w2528:dbl)
    n1775 = Array Size(array=w2446) -> (size(s)=w2534:i32)
    n1776 = Add(x=w2534, y=w2528) -> (x+y=w2529:dbl)
    n1777 = Unbundle By Name(w2329) -> ("Y"=w2327:dbl[])
    n1778 = feedback #3(w2447) -> (w2518:u32[])
    n1779 = Build Array (concatenate)(w2518, w2447) -> (w2515:u32[])
    n1780 = feedback #4(w2392) -> (w2411:u32[])
    n1781 = Divide(x="Bead Sep. Int. Time (s)", y=w2436) -> (x/y=w2325:dbl)
    n1782 = Build Array (concatenate)(w2411, w2392) -> (w2410:u32[])
    n1783 = Greater?(x=w2529, y=w2531) -> (0:w2530:bool)
    n1784 = feedback #5(w2327) -> (w2328:dbl[])
    n1785 = Build Array (concatenate)(w2327, w2328) -> (w2326:dbl[])
    n1786 = Select(t=w2528, s=w2530, f=w2529) -> (s? t:f=w2527:dbl)
    n1787 = feedback-in #2(w2527) -> ()
    n1788 = Array Size(array=w2515) -> (size(s)=w2512:i32)
    n1789 = Array Size(array=w2447) -> (size(s)=w2514:i32)
    n1790 = local read "MCL Scanning"() -> (w2525:bool)
    n1791 = local read "APD Integration Time (s)"() -> (w2419:dbl)
    n1792 = Build Array (concatenate)(w2412, w2551) -> (w2414:waveform(dbl)[])
    "All Signals" <- w2414
    n1793 = Split 1D Array(array=w2326, index=w2325) -> (first subarray=w2319:dbl[])  [unwired: 1 out]
    n1794 = feedback-in #5(w2319) -> ()
    n1795 = Multiply(x=w2514, y="APD Ave N") -> (x*y=w2513:dbl)
    n1796 = Greater?(x=w2512, y=w2513) -> (0:w2516:bool)
    n1797 = Not(x=w2530) -> (.not. x?=w2524:bool)
    n1798 = To Double Precision Float(number=w2392) -> (double precision float=w2391:dbl[])
    n1799 = call-poly <vilib>:"Mean.vi"("X"=w2319) -> ("mean"=w2318:dbl)  [unwired: 1 out]
    "Mean T1 Position (nm)" <- w2318
    n1800 = Subtract(x=w2319, y=w2318) -> (x-y=w2324:dbl[])
    n1801 = Square(x=w2324) -> (x^2=w2323:dbl[])
    n1802 = And(x=w2524, y=w2525) -> (x .and. y?=w2526:bool)
    n1803 = call-poly <vilib>:"Mean.vi"("X"=w2323) -> ("mean"=w2322:dbl)  [unwired: 1 out]
    n1804 = case shown="True" w2516 {
      tunnel: w2515 -> [w2835 w2842]
      tunnel: [w2835 w2840] -> w2463
      tunnel: w2513 -> [_ w2837]
      tunnel: w2512 -> [_ w2841]
      tunnel: w2410 -> [w2834 w2839]
      tunnel: [w2834 w2836] -> w2407
      frame False {
      }
      frame True {
        n1805 = Subtract(x=w2841, y=w2837) -> (x-y=w2838:dbl)
        n1806 = Array Subset(array=w2842, index=w2838, length=w2837) -> (w2840:u32[])
        n1807 = Array Subset(array=w2839, index=w2838, length=w2837) -> (w2836:u32[])
      }
    }
    n1808 = feedback-in #3(w2463) -> ()
    n1809 = feedback-in #4(w2407) -> ()
    n1810 = Or(x=w2526, y=w2522) -> (x .or. y?=w2523:bool)
    n1811 = Square Root(x=w2322) -> (sqrt(x)=w2321:dbl)
    n1812 = Equal?(x="Tab Control 6", y=T36."High Res Display") -> (x = y?=w2453:bool)
    n1813 = Multiply(x="APD Disp. Scale", y=w2412) -> (x*y=w2421:waveform(dbl)[])
    n1814 = Multiply(x="APD Disp. Downsample", y=w2419) -> (x*y=w2417:dbl)
    n1815 = Multiply(x=10.0, y=w2321) -> (x*y=→"Trap 1 Position RMS (A)":dbl)
    n1816 = Divide(x=w2421, y=w2417) -> (x/y=w2389:waveform(dbl)[])
    n1817 = Index Array(array=w2389, index=0) -> (element=w2399:waveform(dbl))
    n1818 = case "For computing FFTs for display" shown="True" "Compute FFT" {
      tunnel: w2416 -> [_ w3519]
      frame False {
      }
      frame True {
        n1819 = Build Array("FFT 1 Choice 1", "FFT 1 Choice 2", "FFT 2 Choice 1", "FFT 2 Choice 2") -> (w3512:u16[])
        n1820 = Array Size(array=w3519) -> (size(s)=w3518:i32)
        n1821 = feedback-in #6(w3512) -> ()
        n1822 = feedback #6(u16[] [100, 100, 100, 100]) -> (w3513:u16[])
        n1823 = feedback-in #7("# Spectra to Ave.") -> ()
        n1824 = feedback #7("# Spectra to Ave.") -> (w3510:dbl)
        n1825 = Not Equal?(x="# Spectra to Ave.", y=w3510) -> (x != y?=w3509:bool)
        n1826 = Not Equal?(x=w3512, y=w3513) -> (x != y?=w3511:bool)
        n1827 = feedback #8(1.0) -> (w3496:dbl)
        n1828 = Compound Arithmetic op=OR("Reset FFT", w3511, w3509) -> (w3494:bool)
        n1829 = Select(t=1.0, s=w3494, f=w3496) -> (s? t:f=w3498:dbl)
        n1830 = Greater?(x=w3498, y="# Spectra to Ave.") -> (0:w3517:bool)
        n1831 = Increment(x=w3498) -> (x+1=w3497:dbl)
        n1832 = feedback-in #8(w3497) -> ()
        n1833 = local read "DMA Update Period (s)"() -> (w3492:dbl)
        n1834 = Multiply(x="# Spectra to Ave.", y=w3492) -> (x*y=→"Ave. Time (s)":dbl)
        n1835 = Build Array(cluster{"f0":dbl, "df":dbl, "magnitude":dbl[]} {"f0"=0.0, "df"=0.0, "magnitude"=[]} ("PSD")) -> (w3501:cluster{"f0":dbl, "df":dbl, "magnitude":dbl[]}[])
        n1836 = Build Array(w3501, w3501, w3501, w3501) -> (w3503:T47)
        n1837 = feedback #9(w3503) -> (w3508:T47)
        n1838 = for {
          N: 4 -> [_]
          tunnel: w3512 -> [w3541] mode=indexing
          tunnel: w3519 -> [w3542]
          tunnel: w3518 -> [w3544]
          tunnel: w3494 -> [w3537]
          tunnel: w3517 -> [w3536]
          tunnel: "# Spectra to Ave." -> [w3535]
          tunnel: [w3534] -> w3507 mode=indexing
          tunnel: w3508 -> [w3539] mode=indexing
          tunnel: [w3538] -> w3495 mode=indexing
          tunnel: w3498 -> [w3533]
          n1839 = Less?(x=w3541, y=w3544) -> (x < y?=w3543:bool)
          n1840 = Index Array(array=w3542, index=w3541) -> (element=w3540:waveform(dbl))
          n1841 = case shown="True" w3543 {
            tunnel: w3540 -> [_ w3561]
            tunnel: w3539 -> [w3546 w3559]
            tunnel: [w3546 w3547] -> w3538
            tunnel: w3537 -> [_ w3558]
            tunnel: w3536 -> [_ w3551]
            tunnel: w3535 -> [_ w3550]
            tunnel: [cluster{"f0":dbl, "df":dbl, "magnitude":dbl[]} {"f0"=0.0, "df"=0.0, "magnitude"=[]} ("PSD") w3552] -> w3534
            tunnel: w3533 -> [_ w3549]
            frame False {
            }
            frame True {
              n1842 = call <vilib>:"Std Deviation and Variance.vi"("X"=w3561) -> ("mean"=w3562:dbl)  [unwired: 1 in, 2 out]
              n1843 = Subtract(x=w3561, y=w3562) -> (x-y=w3560:waveform(dbl))
              n1844 = xnode "Spectral Measurements"("Signals"=w3560) -> ("PSD"=w3554:cluster{"f0":dbl, "df":dbl, "magnitude":dbl[]})  [unwired: 1 in, 1 out]
              n1845 = case shown="False" w3558 {
                tunnel: w3559 -> [w3571 _]
                tunnel: [w3567 w3576] -> w3547
                tunnel: w3554 -> [w3570 w3577]
                tunnel: w3551 -> [w3569 _]
                frame False {
                  n1846 = Build Array (concatenate)(w3571, w3570) -> (w3568:cluster{"f0":dbl, "df":dbl, "magnitude":dbl[]}[])
                  n1847 = case shown="True" w3569 {
                    tunnel: w3568 -> [w3572 w3575]
                    tunnel: [w3572 w3573] -> w3567
                    frame False {
                    }
                    frame True {
                      n1848 = Delete From Array(array=w3575, index=0) -> (array with subset deleted=w3573:cluster{"f0":dbl, "df":dbl, "magnitude":dbl[]}[])  [unwired: 1 in, 1 out]
                    }
                  }
                }
                frame True {
                  n1849 = Build Array(w3577) -> (w3576:cluster{"f0":dbl, "df":dbl, "magnitude":dbl[]}[])
                }
              }
              n1850 = for {
                tunnel: w3547 -> [w3566] mode=indexing
                tunnel: [w3565] -> w3557 mode=indexing
                workers-P: _ -> [_]
                n1851 = Unbundle By Name(w3566) -> ("magnitude"=w3565:dbl[])
              }
              n1852 = Transpose 2D Array(2D array=w3557) -> (transposed array=w3556:dbl[][])
              n1853 = for {
                tunnel: w3556 -> [w3564] mode=indexing
                tunnel: [w3563] -> w3555 mode=indexing
